vi "Generate Message_New Status Log.vi"(7 "QRD":T1, 8 "error in":errorcluster) -> (0 "error out":errorcluster, 2 "Status Log Message":string, 5 "QRD Out":T1)   [LabVIEW 2025]
uses:
  Controls/Queues-Refs-Data.ctl
  Builds/Queue Wrappers.lvlibp/Q Packet.ctl
  Builds/Queue Wrappers.lvlibp
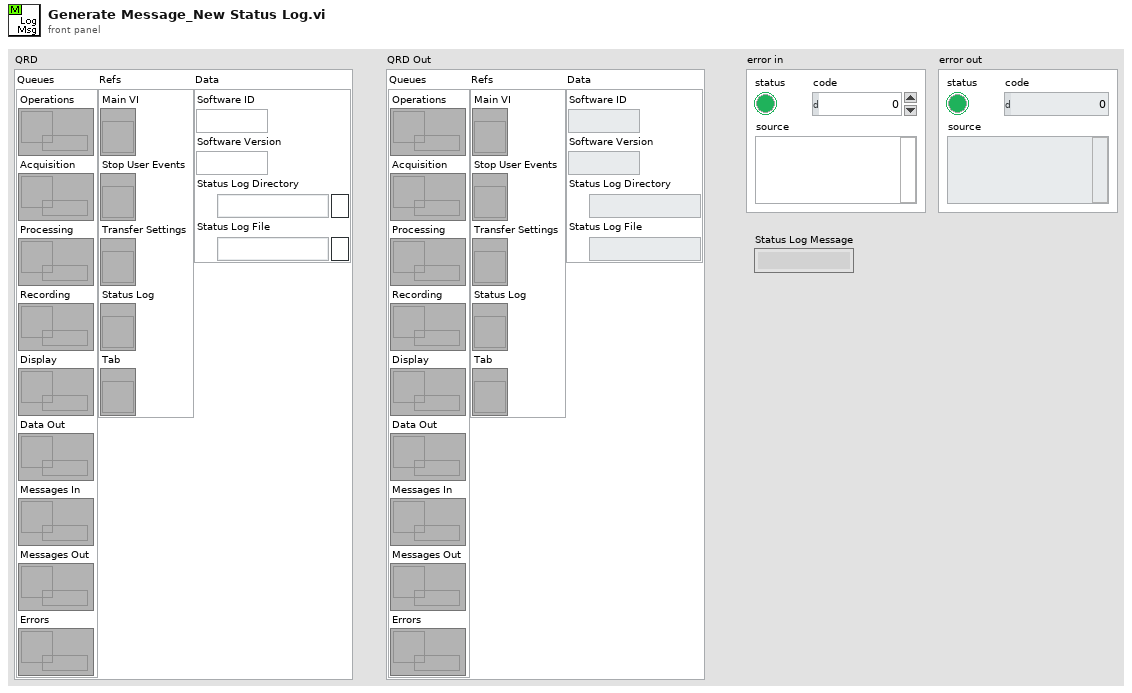
[diagram p1: front panel]
types:
  T1 = typedef "Queues-Refs-Data.ctl" = cluster{"Queues":cluster{"Operations":refnum<queue>, "Acquisition":refnum<queue>, "Processing":refnum<queue>, "Recording":refnum<queue>, "Display":refnum<queue>, "Data Out":refnum<queue>, "Messages In":refnum<queue>, "Messages Out":refnum<queue>, "Errors":refnum<queue>}, "Refs":cluster{"Main VI":refnum<vi>, "Stop User Events":refnum<vi>, "Transfer Settings":refnum<vi>, "Status Log":refnum<vi>, "Tab":refnum<vi>}, "Data":cluster{"Software ID":string, "Software Version":string, "Status Log Directory":path, "Status Log File":path}}
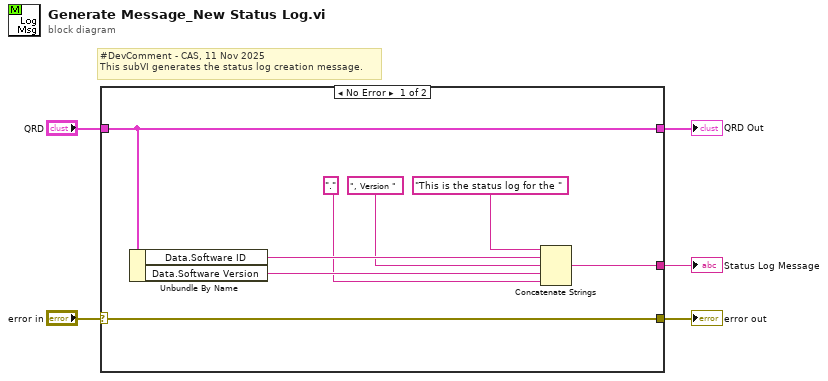
[diagram p0: block diagram]
diagram:
  # "#DevComment - CAS, 11 Nov 2025\nThis subVI generates the status log creation message."
  n1 = case shown="No Error" "error in" {
    selector: "error in" -> [w7 w14]
    tunnel: [w8 _] -> w5
    tunnel: "QRD" -> [w6 w15]
    tunnel: [w7 w14] -> w2
    tunnel: [w6 w15] -> w1
    frame No Error {
      n2 = Unbundle By Name(w6) -> ("Data.Software ID"=w12:string, "Data.Software Version"=w10:string)
      n3 = Concatenate Strings("This is the status log for the " ("string"), w12, ", Version " ("string"), w10, "." ("string")) -> (w8:string)
    }
    frame Error {
    }
  }
  "QRD Out" <- w1
  "error out" <- w2
  "Status Log Message" <- w5
